vi "modulation.vi"(8 "error in":errorcluster, 9 "Symbol Energy":dbl=1.0 format="%#_4p", 10 "input bit stream":u8[](array[numeric]), 11 "Modulation Parameters In":T1 {"TX Parameters"."TX Sample Rate" items=["4M"]}) -> (0 "error out":errorcluster, 2 "Output Symbols":cdb[](array[numeric]), 3 "Modulation Parameters Out":T1 {"TX Parameters"."TX Sample Rate" items=["4M"]})   [LabVIEW 2012]
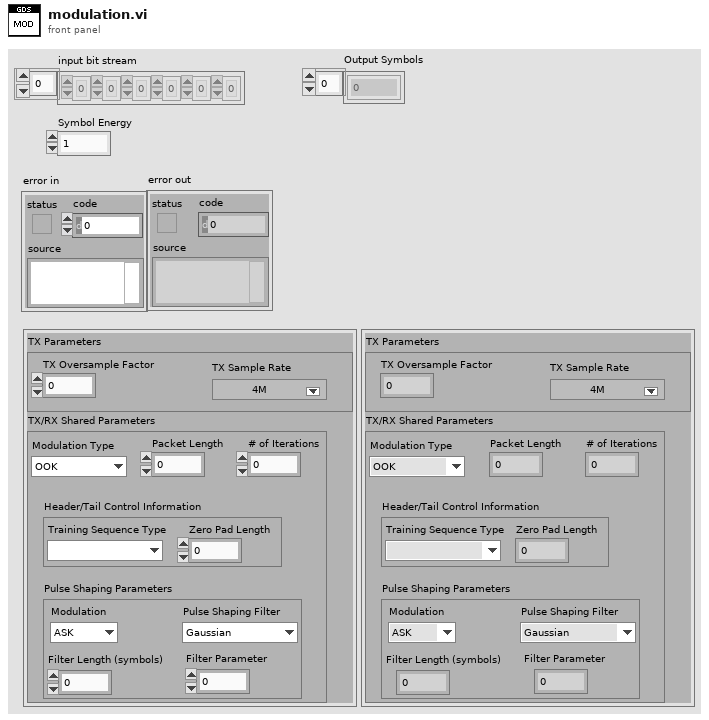
[diagram p1: front panel]
types:
  T1 = cluster{"TX Parameters":cluster{"TX Oversample Factor":u16, "TX Sample Rate":dbl}, "TX/RX Shared Parameters":cluster{"Modulation Type":enum16{"OOK", "FSK"}, "Packet Length":dbl, "# of Iterations":dbl, "Pulse Shaping Parameters":cluster{"Modulation":enum16{"ASK", "FSK", "PSK", "QAM", "MSK", "PAM"}, "Pulse Shaping Filter":enum16{"Gaussian"}, "Filter Length (symbols)":dbl, "Filter Parameter":dbl}, "Header/Tail Control Information":cluster{"Training Sequence Type":enum16{""}, "Zero Pad Length":dbl}}}
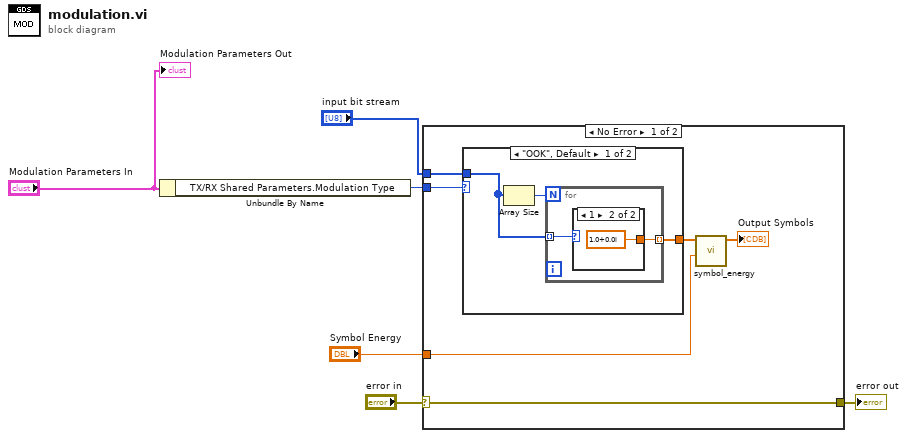
[diagram p0: block diagram]
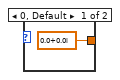
[diagram p2: hidden frame]
diagram:
  n1 = Unbundle By Name("Modulation Parameters In") -> ("TX/RX Shared Parameters.Modulation Type"=w5:enum16{"OOK", "FSK"})
  n2 = case shown="No Error" "error in" {
    selector: "error in" -> [w8 w21]
    tunnel: w5 -> [w12 _]
    tunnel: "input bit stream" -> [w11 _]
    tunnel: [w8 w21] -> w3
    tunnel: "Symbol Energy" -> [w7 _]
    frame No Error {
      n3 = case shown="\"OOK\", Default" w12 {
        tunnel: w11 -> [w15 w20]
        tunnel: [w13 w20] -> w10
        frame "OOK", Default {
          n4 = Array Size(array=w15) -> (size(s)=w14:i32)
          n5 = for {
            N: w14 -> [_]
            tunnel: w15 -> [w17] mode=indexing
            tunnel: [w16] -> w13 mode=indexing
            n6 = case shown="1" w17 {
              tunnel: [cdb 0.0+0.0i cdb 1.0+0.0i] -> w16
              frame 0, Default {
              }
              frame 1 {
              }
            }
          }
        }
        frame "FSK" {
        }
      }
      n7 = call "symbol_energy.vi"("Symbol Energy"=w7, "Input Symbols"=w10) -> ("Output Symbols"=→"Output Symbols":cdb[])  [unwired: 9 in]
    }
    frame Error {
    }
  }
  "error out" <- w3
  "Modulation Parameters Out" <- "Modulation Parameters In"
